vi "Set Image.vi"(8 "error in (no error)":errorcluster, 10 "Image in":T2, 11 "Item Ref in":T1 format="%.0x") -> (0 "error out":errorcluster, 2 "Image out":T2, 3 "Item Ref out":T1 format="%.0x")   [LabVIEW 2011, in "Meter Detection Custom Device.lvlib"]
uses:
  Meter Detection Custom Device.lvlib
  <vilib>/vision/Image Controls.llb/IMAQ Image.ctl
  <vilib>/NI Veristand/Custom Device API/Custom Device Item Ref.ctl
  Meter Detection Global Variable.vi
  <vilib>/NI Veristand/Custom Device API/Set Item Property (Variant).vi
  <vilib>/NI Veristand/Custom Device API/Custom Device API.lvlib
  <vilib>/vision/NI_Vision_Development_Module.lvlib
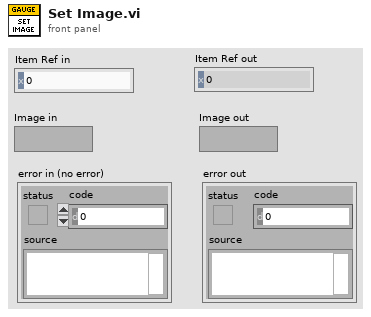
[diagram p1: front panel]
types:
  T1 = typedef "Custom Device API.lvlib/Custom Device Item Ref.ctl" = u64
  T2 = typedef "IMAQ Image.ctl" = refnum<image>
  T3 = typedef "Image Type" = u32
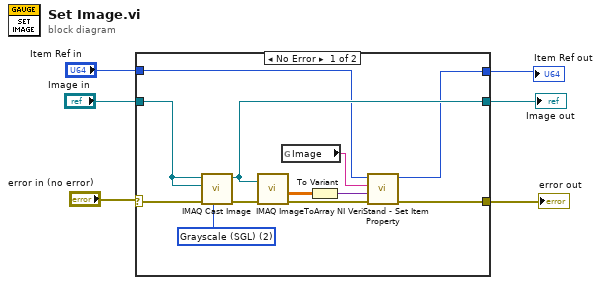
[diagram p0: block diagram]
diagram:
  n1 = case shown="No Error" "error in (no error)" {
    selector: "error in (no error)" -> [w7 w19]
    tunnel: [w18 w20] -> w6
    tunnel: "Image in" -> [w17 w20]
    tunnel: [w11 w19] -> w4
    tunnel: "Item Ref in" -> [w10 w21]
    tunnel: [w8 w21] -> w2
    frame No Error {
      w15 = T3 2 items=["Grayscale (U8)", "Grayscale (I16)", "Grayscale (SGL)", "Complex (CSG)", "RGB (U32)", "HSL (U32)", "RGB (U64)", "Grayscale (U16)"] ("Image Type")
      n2 = call "IMAQ Cast Image"("Image Type"=w15, "error in (no error)"=w7, "Image Dst"=w17, "Image Src"=w17) -> ("error out"=w16:errorcluster, "Image Dst Out"=w18:T2)  [unwired: 6 in]
      n3 = call "IMAQ ImageToArray"("error in (no error)"=w16, "Image"=w18) -> ("Image Pixels (Float)"=w14:sgl[][], "error out"=w13:errorcluster)  [unwired: 2 in, 3 out]
      n4 = global read "Meter Detection Global Variable.vi" "Image"() -> (w12:string)
      n5 = To Variant(anything=w14) -> (Variant=w9:variant)
      n6 = call-poly <vilib>:"NI VeriStand - Set Item Property.vi"("error in (no error)"=w13, "Value"=w9, "Property Name"=w12, "Item Ref in"=w10) -> ("error out"=w11:errorcluster, "Item Ref out"=w8:T1)  [unwired: 5 in, 1 out]
    }
    frame Error {
    }
  }
  "Image out" <- w6
  "error out" <- w4
  "Item Ref out" <- w2
